vi "Clean.vi"(8 "error in (no error)":errorcluster, 11 "Tamagotchi Full Actor in":refnum<class "Tamagotchi Full Actor.lvclass">) -> (0 "error out":errorcluster, 3 "Tamagotchi Full Actor out":refnum<class "Tamagotchi Full Actor.lvclass">)   [LabVIEW 2026, in "Tamagotchi Full Actor.lvclass"]
uses:
  Tamagotchi Full Actor.lvclass
  Tamagotchi Full Actor.lvclass/Tamagotchi Full Actor.ctl
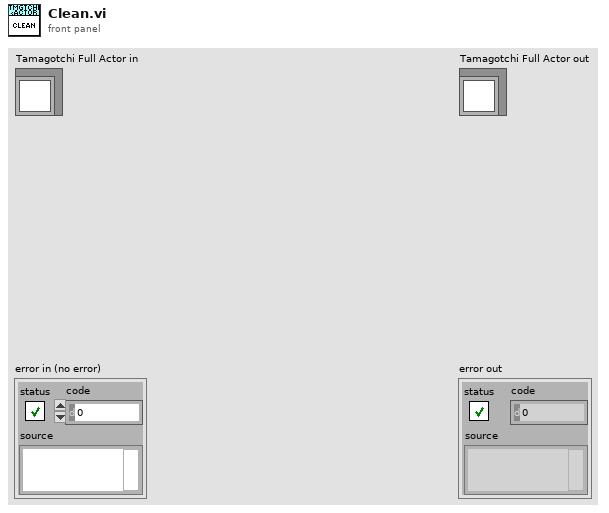
[diagram p1: front panel]
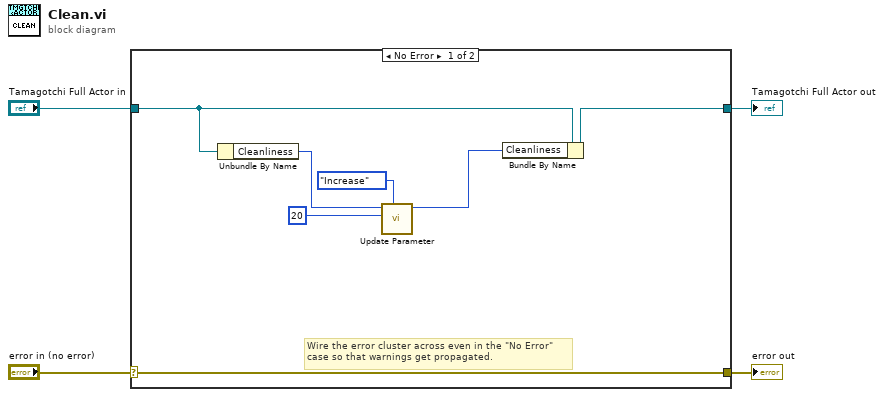
[diagram p0: block diagram]
diagram:
  n1 = case shown="No Error" "error in (no error)" {
    selector: "error in (no error)" -> [w11 w13]
    tunnel: [w11 w13] -> w3
    tunnel: [w5 w12] -> w1
    tunnel: "Tamagotchi Full Actor in" -> [w6 w12]
    frame No Error {
      # "Wire the error cluster across even in the \"No Error\"\ncase so that warnings get propagated."
      n2 = Unbundle By Name(w6) -> ("Cleanliness"=w9:i16)
      n3 = call "Update Parameter.vi"("Action"=enum16{"Increase", "Decrease"}."Increase", "Modifier"=i16 20 ("y"), "Parameter"=w9) -> ("New Value"=w10:i16)  [unwired: 8 in]
      n4 = Bundle By Name(cluster=w6, "Cleanliness"=w10) -> (w5:refnum<class "Tamagotchi Full Actor.lvclass">)
    }
    frame Error {
    }
  }
  "error out" <- w3
  "Tamagotchi Full Actor out" <- w1
